vi "Reference To UID.vi"(11 "Reference":refnum<vi>) -> (3 "UID":i32)   [LabVIEW 2014]
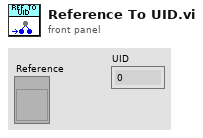
[diagram p1: front panel]
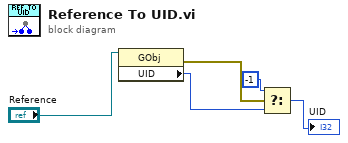
[diagram p0: block diagram]
diagram:
  n1 = property class="GObj"(reference="Reference") -> (error out=w4:errorcluster, "UID"=w2:i32)  [unwired: 1 in, 1 out]
  n2 = Select(t=-1, s=w4, f=w2) -> (s? t:f=→"UID":i32)
